vi "CTRE_CANifier_ConfigVelocityMeasurementWindow.vi"(6 "timeoutMs":i32, 8 "error in":errorcluster, 10 "windowSize":i32=1, 11 "CANifierDevRef":T1) -> (0 "error out":errorcluster, 3 "CANifierDevRef":T1)   [LabVIEW 2020]
uses:
  <vilib>/Rock Robotics/WPI/ThirdParty/Phoenix-LabVIEW/CANifier/CTRE_CANifier_DeviceRef.ctl
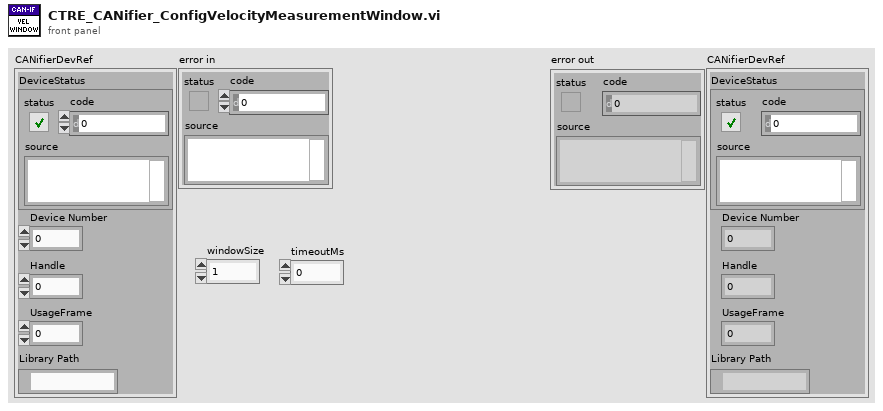
[diagram p1: front panel]
types:
  T1 = typedef "CTRE_CANifier_DeviceRef.ctl" = cluster{"DeviceStatus":errorcluster, "Device Number":u8, "Handle":u64, "UsageFrame":u32, "Library Path":path}
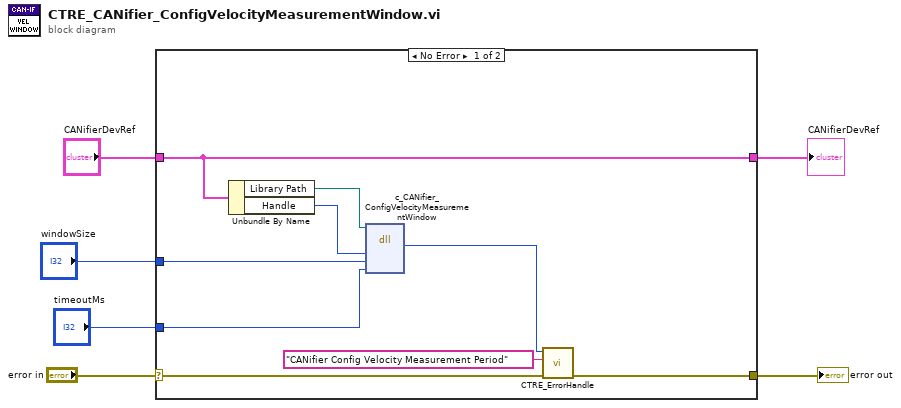
[diagram p0: block diagram]
diagram:
  n1 = case shown="No Error" "error in" {
    selector: "error in" -> [w12 w17]
    tunnel: "CANifierDevRef" -> [w13 w16]
    tunnel: [w11 w17] -> w4
    tunnel: [w13 w16] -> w3
    tunnel: "timeoutMs" -> [w8 _]
    tunnel: "windowSize" -> [w7 _]
    frame No Error {
      n2 = Unbundle By Name(w13) -> ("Library Path"=w15:path, "Handle"=w14:u64)
      n3 = dll-call lib="?" fn="c_CANifier_ConfigVelocityMeasurementWindow"(path in=w15, "handle"=w14, "window"=w7, "timeoutMs"=w8) -> ("CTR_Code"=w10:i8)  [unwired: 5 in, 2 out]
      n4 = call <vilib>:"CTRE_ErrorHandle.vi"("error in"=w12, "origin"="CANifier Config Velocity Measurement Period", "code"=w10) -> ("error out"=w11:errorcluster)  [unwired: 8 in]
    }
    frame Error {
    }
  }
  "error out" <- w4
  "CANifierDevRef" <- w3
